vi "P7.vi"() -> ()   [LabVIEW 2024]
panel:
  out "Temp":dbl(slide) scale=0.0..100.0
  out "Mj , mv":dbl
  out "Vdiff, mv":dbl format="%0#1.3f"
  out "Vcc, V":dbl format="%0#1.3f"
  out "AtoD":i32 format="%04x"
  in  "stop":bool
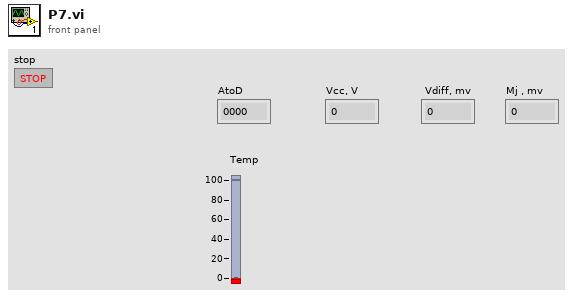
[diagram p1: front panel]
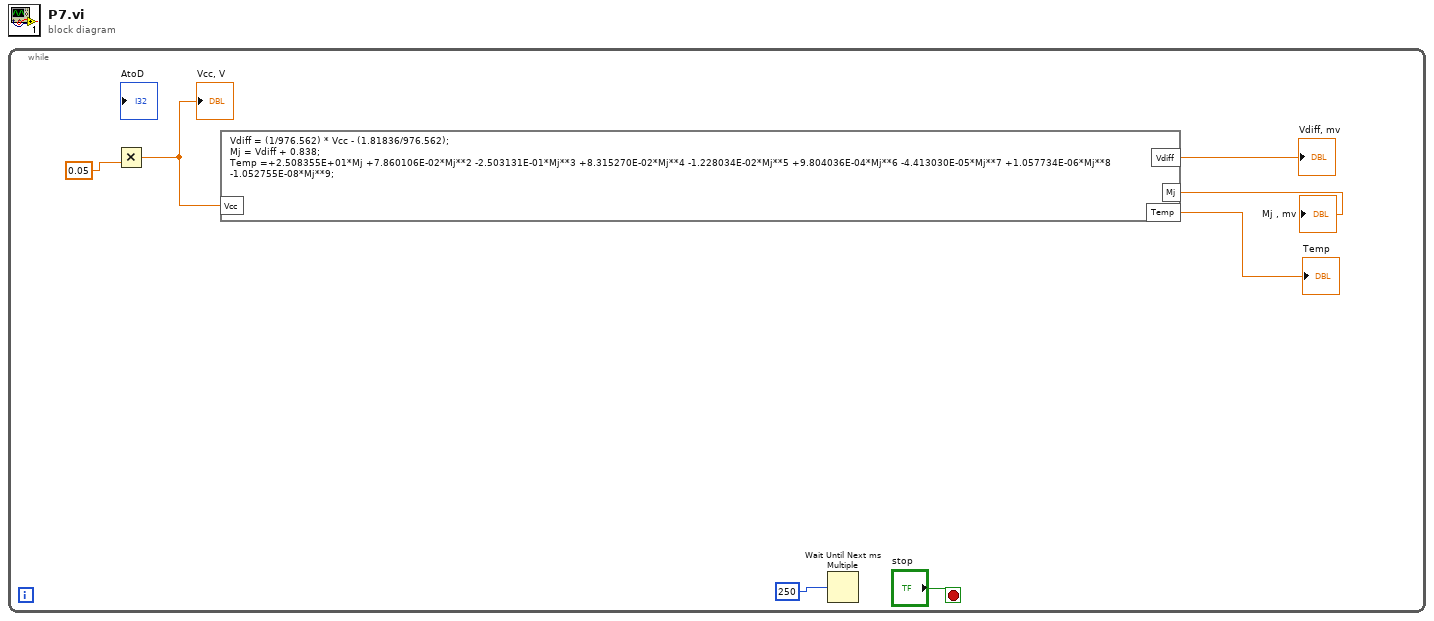
[diagram p0: block diagram]
diagram:
  n1 = while {
    stop <- "stop" stop-if-true
    n2 = Multiply(y=0.05) -> (x*y=w4:dbl)  [unwired: 1 in]
    "Vcc, V" <- w4
    n3 = formula code="Vdiff = (1/976.562) * Vcc - (1.81836/976.562);\nMj = Vdiff + 0.838;\nTemp =+2.508355E+01*Mj +7.860106E-02*Mj**2 -2.503131E-01*Mj**3 +8.315270E-02*Mj**4 -1.228034E-02*Mj**5 +9.804036E-04*Mj**6 -4.413030E-05*Mj**7 +1.057734E-06*Mj**8 -1.052755E-08*Mj**9;"("Vcc"=w4) -> ("Vdiff"=→"Vdiff, mv":dbl, "Mj"=→"Mj , mv":dbl, "Temp"=→"Temp":dbl)
    n4 = Wait Until Next ms Multiple(millisecond multiple=250) -> ()  [unwired: 1 out]
  }
